vi "set value of int32 pointer.vi"(8 "error in (no error)":errorcluster, 10 "value (0)":i32, 11 "pointer in":u64) -> (0 "error out":errorcluster, 3 "pointer out":u64)   [LabVIEW 2013, in "Linux Errno.lvlib"]
uses:
  Linux Errno.lvlib
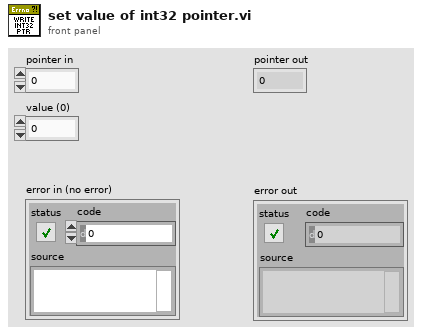
[diagram p1: front panel]
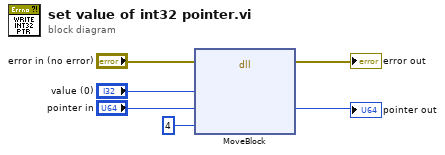
[diagram p0: block diagram]
diagram:
  n1 = dll-call lib="LabVIEW" fn="MoveBlock"(error in="error in (no error)", "data"="value (0)", "pointer"="pointer in", "size"=u64 4) -> (error out=→"error out":errorcluster, "pointer"=→"pointer out":u64)  [unwired: 5 in, 1 out]
